vi "pre-allocated_no_IPE.vi"(8 "error in (no error)":errorcluster, 10 "data bus in":T1, 11 "Test Data in":T2) -> (0 "error out":errorcluster, 2 "data bus out":T1, 3 "Test Data out":T2)   [LabVIEW 2024, in "IPE Optimization Tester.lvlib"]
uses:
  IPE Optimization Tester.lvlib
  test_data--cluster.ctl
  SubVIs/data_bus--cluster.ctl
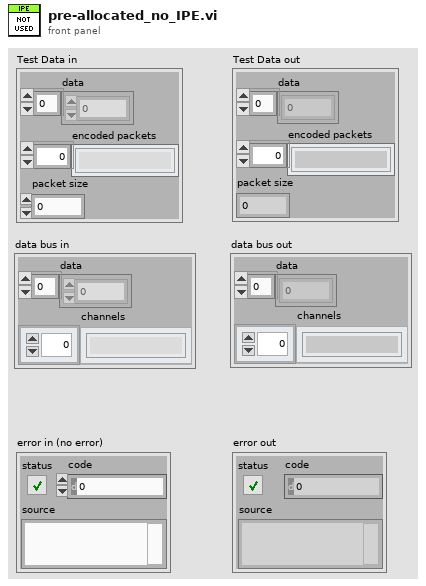
[diagram p1: front panel]
types:
  T1 = typedef "IPE Optimization Tester.lvlib/data_bus--cluster.ctl" = cluster{"data":dbl[], "channels":string[]}
  T2 = typedef "IPE Optimization Tester.lvlib/test_data--cluster.ctl" = cluster{"data":dbl[], "encoded packets":string[], "packet size":i32}
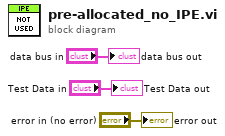
[diagram p0: block diagram]
diagram:
  "Test Data out" <- "Test Data in"
  "error out" <- "error in (no error)"
  "data bus out" <- "data bus in"
